vi "FMPA Set up E-712 data recorder - Double HexNano, 11 Aug 17.vi"(5 "Step axis sensor ch":string, 7 "Scan axis sensor ch":string, 8 "error in":errorcluster, 9 "Table rate":i32=10, 10 "Opt. Ch.":i32=10, 11 "System no.":i32) -> (0 "error out":errorcluster)   [LabVIEW 2023]
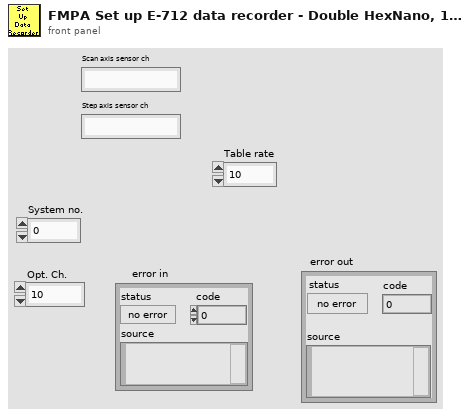
[diagram p1: front panel]
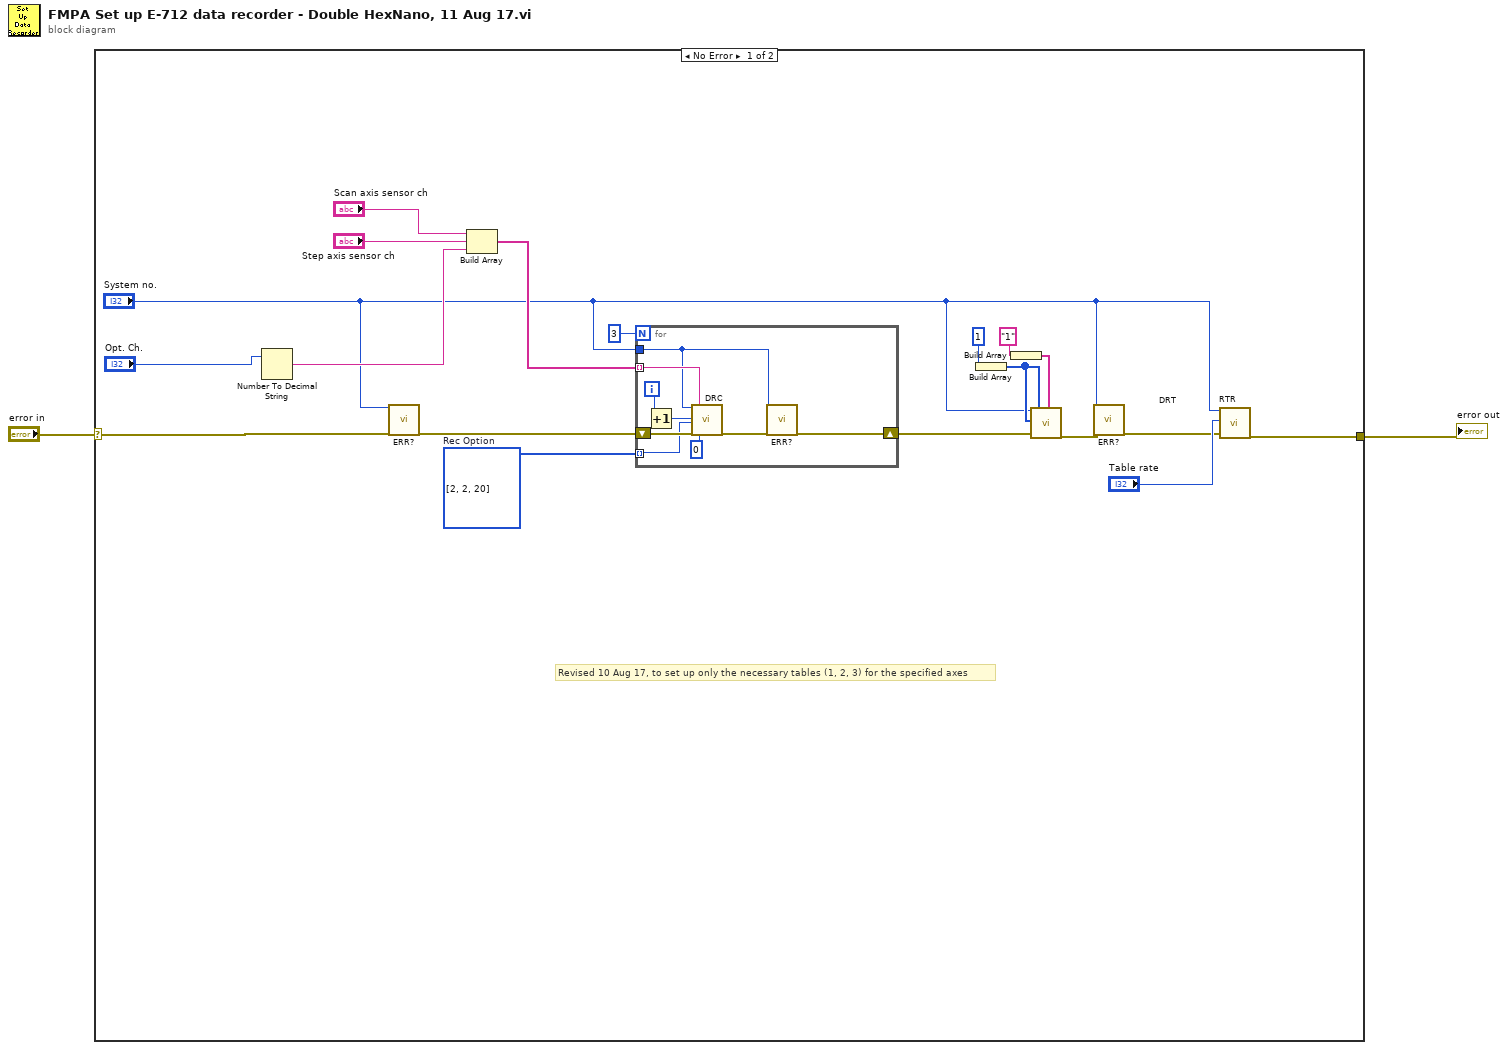
[diagram p0: block diagram]
diagram:
  n1 = case shown="No Error" "error in" {
    selector: "error in" -> [w7 w31]
    tunnel: [w21 w31] -> w1
    frame No Error {
      w11 = i32[] [2, 2, 20]  # Rec Option
      # "Revised 10 Aug 17, to set up only the necessary tables (1, 2, 3) for the specified axes"
      n2 = Number To Decimal String(number="Opt. Ch.") -> (decimal integer string=w20:string)  [unwired: 1 in]
      n3 = call "ERR?.vi"("System no."="System no.", "error in"=w7) -> ("error out"=w6:errorcluster)  [unwired: 16 in, 1 out]
      n4 = Build Array("Scan axis sensor ch", "Step axis sensor ch", w20) -> (w13:string[])
      n5 = for {
        N: 3 -> [_]
        shift-right: [w22] -> w19
        shift-left: w6 -> [w30]
        tunnel: "System no." -> [w23]
        tunnel: w11 -> [w28] mode=indexing
        tunnel: w13 -> [w25] mode=indexing
        i -> [w29]
        n6 = Increment(x=w29) -> (x+1=w27:i32)
        n7 = call "DRC.vi"("System no."=w23, "Rec. table"=w27, "Rec. option"=w28, "error in"=w30, "Source ID"=w25, "Trigger option"=0) -> ("error out"=w24:errorcluster)  [unwired: 13 out]
        n8 = call "ERR?.vi"("System no."=w23, "error in"=w24) -> ("error out"=w22:errorcluster)  [unwired: 16 in, 1 out]
      }
      n9 = Build Array(1) -> (w17:i32[])
      n10 = Build Array("1") -> (w15:string[])
      n11 = call "DRT.vi"("System no."="System no.", "DataRecorderTable"=w17, "error in"=w19, "Trigger source"=w17, "Value"=w15) -> ("error out"=w5:errorcluster)  [unwired: 14 out]
      n12 = call "ERR?.vi"("System no."="System no.", "error in"=w5) -> ("error out"=w3:errorcluster)  [unwired: 16 in, 1 out]
      n13 = call "RTR.vi"("System no."="System no.", "Table rate"="Table rate", "error in"=w3) -> ("error out"=w21:errorcluster)  [unwired: 16 out]
    }
    frame Error {
    }
  }
  "error out" <- w1
